vi "Update Changed Edges.vi"(10 "WorldMapEdge":T1, 11 "AD* in":refnum<class "NI_Robotics_AnytimeDStar.lvclass">) -> (2 "updated":bool, 3 "AD* out":refnum<class "NI_Robotics_AnytimeDStar.lvclass">)   [LabVIEW 2017, in "NI_Robotics_AnytimeDStar.lvclass"]
uses:
  <vilib>/robotics/Navigation/Anytime D Star/NI_Robotics_AnytimeDStar.lvclass
  <vilib>/robotics/Navigation/shared/WorldMap/World Map Edge.ctl
  <vilib>/robotics/Navigation/shared/MapNode/AbstractMapNode/NI_Robotics_AbstractMapNode.lvclass
  <vilib>/robotics/Navigation/Anytime D Star/NI_Robotics_AnytimeDStar.lvclass/NI_Robotics_AnytimeDStar.ctl
  <vilib>/robotics/Navigation/shared/MapNode/AbstractDstarNode/NI_Robotics_AbstractDstarNode.lvclass
  c:/Program Files (x86)/National Instruments/LabVIEW 2017/vi.lib/robotics/Navigation/shared/MapNode/AbstractMapNode/NI_Robotics_AbstractMapNode.lvclass
  <vilib>/robotics/Navigation/shared/WorldMap/AbstractWorldMap/NI_Robotics_AbstractWorldMap.lvclass
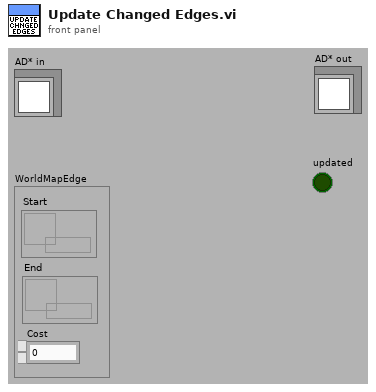
[diagram p1: front panel]
types:
  T1 = typedef "NI_Robotics_AbstractWorldMap.lvclass/World Map Edge.ctl" = cluster{"Start":refnum<data-value>, "End":refnum<data-value>, "Cost":dbl}
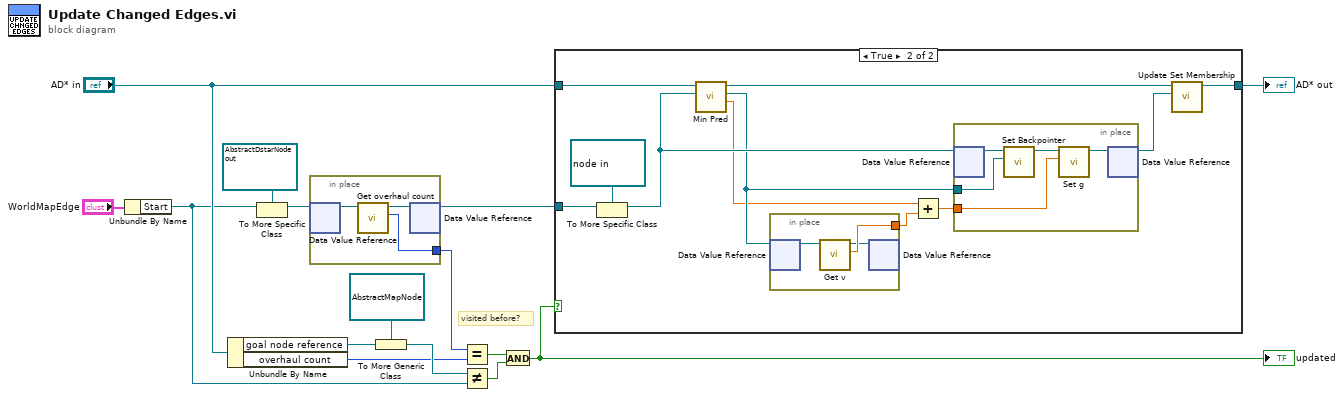
[diagram p0: block diagram]
diagram:
  # "visited before?"
  n1 = Unbundle By Name("WorldMapEdge") -> ("Start"=w8:refnum<data-value>)
  n2 = Unbundle By Name("AD* in") -> ("goal node reference"=w7:refnum<data-value>, "overhaul count"=w5:i32)
  n3 = To More Specific Class(target class=refnum<data-value> refnum ("data value reference"), reference=w8) -> (specific class reference=w3:refnum<data-value>)  [unwired: 1 in, 1 out]
  n4 = in-place {
    in-place-border: [w18] -> w6
    n5 = in-place-dvr #1(w3) -> (w17:refnum<class "NI_Robotics_AbstractDstarNode.lvclass">)  [unwired: 1 out]
    n6 = call <vilib>:"Get overhaul count.vi"("AbstractDstarNode in"=w17) -> ("overhaul count"=w18:i32, "AbstractDstarNode out"=w16:refnum<class "NI_Robotics_AbstractDstarNode.lvclass">)  [unwired: 9 in]
    n7 = in-place-dvr #1(w16) -> (w2:refnum<data-value>)  [unwired: 1 out]
  }
  n8 = To More Generic Class(target class=refnum<data-value> refnum ("Start"), reference=w7) -> (generic class reference=w14:refnum<data-value>)
  n9 = Equal?(x=w6, y=w5) -> (x = y?=w4:bool)
  n10 = Not Equal?(x=w14, y=w8) -> (x != y?=w12:bool)
  n11 = And(x=w4, y=w12) -> (x .and. y?=w1:bool)
  "updated" <- w1
  n12 = case shown="True" w1 {
    tunnel: "AD* in" -> [w19 w30]
    tunnel: w2 -> [_ w24]
    tunnel: [w19 w26] -> w10
    frame False {
    }
    frame True {
      n13 = To More Specific Class(target class=refnum<data-value> refnum ("node ref in"), reference=w24) -> (specific class reference=w29:refnum<data-value>)  [unwired: 1 in, 1 out]
      n14 = call <vilib>:"Min Pred.vi"("node ref in"=w29, "AD* in"=w30) -> ("cost of node to min pred"=w21:dbl, "min node ref"=w23:refnum<data-value>, "AD* out"=w27:refnum<class "NI_Robotics_AnytimeDStar.lvclass">)  [unwired: 6 in, 1 out]
      n15 = in-place {
        in-place-border: [w33] -> w22
        n16 = in-place-dvr #2(w23) -> (w32:refnum<class "NI_Robotics_AbstractDstarNode.lvclass">)  [unwired: 1 out]
        n17 = call <vilib>:"Get v.vi"("AbstractDstarNode in"=w32) -> ("v"=w33:dbl, "AbstractDstarNode out"=w31:refnum<class "NI_Robotics_AbstractDstarNode.lvclass">)  [unwired: 9 in]
        n18 = in-place-dvr #2(w31) -> ()  [unwired: 2 out]
      }
      n19 = Add(x=w21, y=w22) -> (x+y=w20:dbl)
      n20 = in-place {
        in-place-border: w23 -> [w38]
        in-place-border: w20 -> [w34]
        n21 = in-place-dvr #3(w29) -> (w37:refnum<class "NI_Robotics_AbstractDstarNode.lvclass">)  [unwired: 1 out]
        n22 = call <vilib>:"Set Backpointer.vi"("BackPointer"=w38, "AbstractDstarNode in"=w37) -> ("AbstractDstarNode out"=w36:refnum<class "NI_Robotics_AbstractDstarNode.lvclass">)  [unwired: 8 in, 1 out]
        n23 = call <vilib>:"Set g.vi"("g"=w34, "AbstractDstarNode in"=w36) -> ("AbstractDstarNode out"=w35:refnum<class "NI_Robotics_AbstractDstarNode.lvclass">)  [unwired: 9 in]
        n24 = in-place-dvr #3(w35) -> (w28:refnum<data-value>)  [unwired: 1 out]
      }
      n25 = call <vilib>:"Update Set Membership.vi"("node ref in"=w28, "AD* in"=w27) -> ("AD* out"=w26:refnum<class "NI_Robotics_AnytimeDStar.lvclass">)  [unwired: 8 in, 1 out]
    }
  }
  "AD* out" <- w10
